vi "SubVI_Res_pass-fail.vi"(10 "Current Cycle":i32, 11 "pass/fail":bool[](array[boolean])) -> (2 "Test Stop?":T1, 3 "Fail array":bool[](array[boolean]))   [LabVIEW 2016]
uses:
  Ctrls/Fail flags.ctl
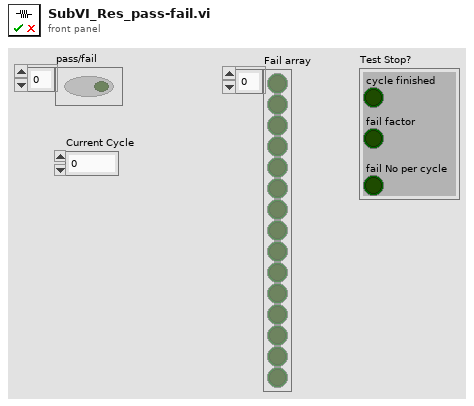
[diagram p1: front panel]
types:
  T1 = typedef "Fail flags.ctl" = cluster{"cycle finished":bool, "fail factor":bool, "fail No per cycle":bool}
  T2 = cluster{"Test Information":cluster{"date":string, "custom":string, "oper":string, "package":string, "pkg side":string, "solder":string, "brd side":string, "paste":string, "reflow":string}, "Sensor Set":cluster{"Accelerometer":cluster{"Sensitivity(mV/g)":dbl}, "Strain Guage":cluster{"Ch.":dbl[], "Gage factor":dbl[], "Resistance":dbl[], "Poisson ratio":dbl[]}}, "Resistor Set":cluster{"Criterion Level":dbl, "Res. Set":cluster{"Res. Ch":dbl, "Res. Active":bool, "Res Initial":dbl}[]}, "Test Stop Condition":cluster{"Test cycle":u16, "Fail number in a cycle":u16, "Fail factor":cluster{"Duration":u16, "Fail No.":u16}}, "Acceleration Condition ":cluster{"Shock duration pecent [%]":u16, "Filter cutoff freq":u32}, "Save":cluster{"Save Path":path, "File Name":string}}
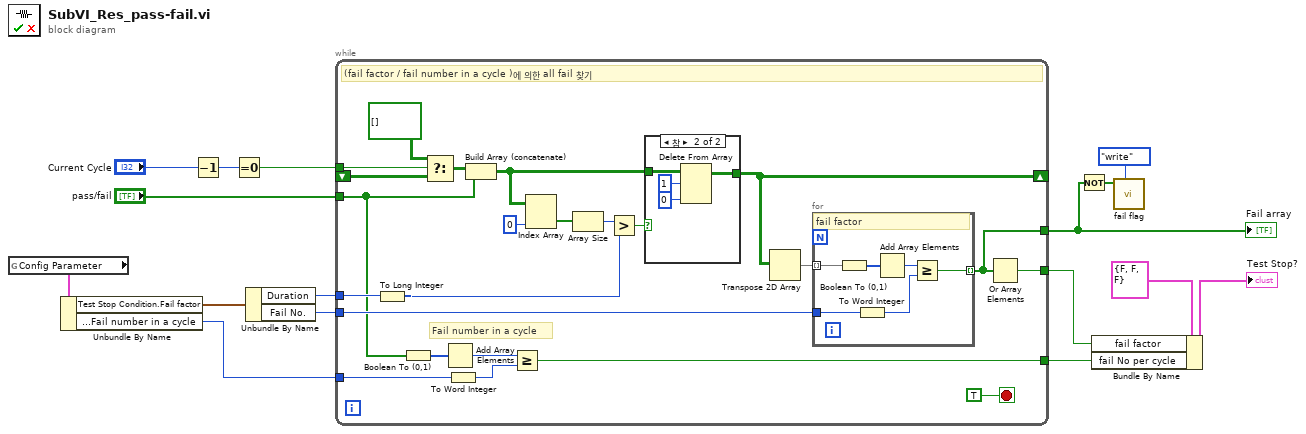
[diagram p0: block diagram]
diagram:
  n1 = global read "글로벌_Config Parameter.vi" "Config Parameter"() -> (w13:T2)
  n2 = Unbundle By Name(w13) -> ("Test Stop Condition.Fail factor"=w6:cluster{"Duration":u16, "Fail No.":u16}, "Test Stop Condition.Fail number in a cycle"=w9:u16)
  n3 = Decrement(x="Current Cycle") -> (x-1=w14:i32)
  n4 = Equal To 0?(x=w14) -> (x = 0?=w16:bool)
  n5 = Unbundle By Name(w6) -> ("Duration"=w7:u16, "Fail No."=w8:u16)
  n6 = while {
    shift-right: [w34] -> _
    shift-left: _ -> [w29]
    tunnel: "pass/fail" -> [w25]
    tunnel: w7 -> [w32]
    tunnel: w8 -> [w30]
    tunnel: w9 -> [w24]
    tunnel: [w20] -> w12
    tunnel: [w19] -> w11
    tunnel: w16 -> [w18]
    tunnel: [w17] -> w1
    stop <- TRUE stop-if-true
    # "Fail number in a cycle"
    # "(fail factor / fail number in a cycle )에 의한 all fail 찾기"
    n7 = To Long Integer(number=w32) -> (32bit integer=w26:i32)
    n8 = Boolean To (0,1)(Boolean=w25) -> (0, 1=w21:i16[])
    n9 = Select(t=bool[][] [] ("ok/ng"), s=w18, f=w29) -> (s? t:f=w28:bool[][])
    n10 = Add Array Elements(numeric array=w21) -> (sum=w23:i16)
    n11 = To Word Integer(number=w24) -> (16bit integer=w22:i16)
    n12 = Build Array (concatenate)(w28, w25) -> (w39:bool[][])
    n13 = Greater Or Equal?(x=w23, y=w22) -> (x >= y?=w20:bool)
    n14 = Index Array(array=w39, index (col)=0 ("disabled index (col)")) -> (element=w37:bool[])  [unwired: 1 in]
    n15 = Array Size(array=w37) -> (size(s)=w36:i32)
    n16 = Greater?(x=w36, y=w26) -> (0:w35:bool)
    n17 = case shown="참" w35 {
      tunnel: w39 -> [w46 w50]
      tunnel: [w46 w48] -> w34
      frame False {
      }
      frame True {
        n18 = Delete From Array(array=w50, length=1, index (row)=0) -> (array with subset deleted=w48:bool[][])  [unwired: 1 in, 1 out]
      }
    }
    n19 = Transpose 2D Array(2D array=w34) -> (transposed array=w33:bool[][])
    n20 = for {
      tunnel: w33 -> [w45] mode=indexing
      tunnel: w30 -> [w42]
      tunnel: [w41] -> w17 mode=indexing
      # "fail factor"
      n21 = Boolean To (0,1)(Boolean=w45) -> (0, 1=w44:i16[])
      n22 = To Word Integer(number=w42) -> (16bit integer=w40:i16)
      n23 = Add Array Elements(numeric array=w44) -> (sum=w43:i16)
      n24 = Greater Or Equal?(x=w43, y=w40) -> (x >= y?=w41:bool)
    }
    n25 = Or Array Elements(Boolean array=w17) -> (logical OR=w19:bool)
  }
  "Fail array" <- w1
  n26 = Not(x=w1) -> (.not. x?=w2:bool[])
  n27 = Bundle By Name(cluster=T1 {"cycle finished"=FALSE, "fail factor"=FALSE, "fail No per cycle"=FALSE} ("Test Stop? 2"), "fail factor"=w11, "fail No per cycle"=w12) -> (→"Test Stop?":T1)
  n28 = call "fail flag.vi"("Command"=enum16{"init", "read", "write"}."write", "Fail Index"=w2) -> ()  [unwired: 9 in, 1 out]
